vi "setPosition_fw103_wait.vi"(8 "waitTimeout":i32=500, 9 "Set position\n(deg) (float)":dbl, 11 "Method reference input":refnum<k24>) -> (1 "Current position (deg) (float)":i32 format="%.3f", 2 "error out":errorcluster, 3 "Method reference out":refnum<k24>)   [LabVIEW 2020]
uses:
  C:/Users/OPMuser/Documents/labview/fw103/Thorlabs.MotionControl.Benchtop.StepperMotorCLI.dll
  Thorlabs.MotionControl.Benchtop.StepperMotorCLI.dll
  <vilib>/Utility/error.llb/Error Cluster From Error Code.vi
  <vilib>/ErrorRing/Error Ring.xnode
panel:
  # "Move filter wheel VI"
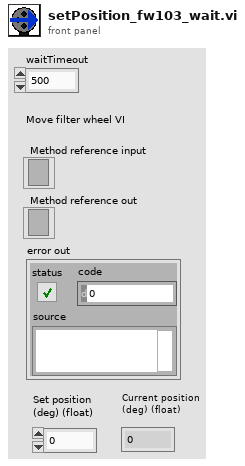
[diagram p1: front panel]
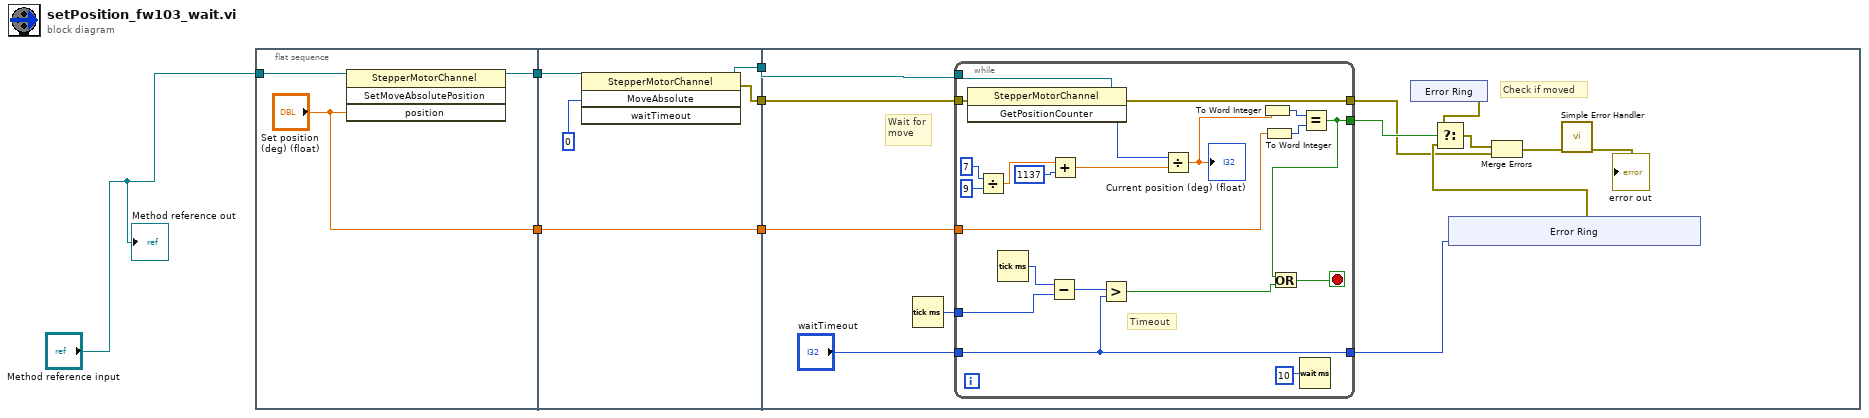
[diagram p0: block diagram]
diagram:
  n1 = flat-sequence {
    tunnel: [w9] -> w6
    tunnel: ["Set position\n(deg) (float)"] -> w3
    tunnel: "Method reference input" -> [w7]
    tunnel: w6 -> [w13]
    tunnel: [w12] -> w5
    tunnel: [w11] -> w4
    tunnel: w3 -> [w11]
    tunnel: [w10] -> w1
    tunnel: w1 -> [w19]
    tunnel: w4 -> [w21]
    tunnel: w5 -> [w22]
    frame #0 {
      n2 = invoke class="StepperMotorChannel" method="SetMoveAbsolutePosition"(reference=w7, "position"="Set position\n(deg) (float)") -> (reference out=w9:refnum<k24>)  [unwired: 2 in, 3 out]
    }
    frame #1 {
      n3 = invoke class="StepperMotorChannel" method="MoveAbsolute"(reference=w13, "waitTimeout"=0) -> (reference out=w12:refnum<k24>, error out=w10:errorcluster)  [unwired: 2 in, 2 out]
    }
    frame #2 {
      # "Wait for\nmove"
      # "Check if moved"
      n4 = Tick Count (ms)() -> (millisecond timer value=w17:u32)
      n5 = while {
        tunnel: w22 -> [w47]
        tunnel: w21 -> [w39]
        tunnel: [w29] -> w20
        tunnel: w19 -> [w35]
        tunnel: [w34] -> w18
        tunnel: w17 -> [w32]
        tunnel: "waitTimeout" -> [w30]
        tunnel: [w30] -> w15
        stop <- w27 stop-if-true
        # "Timeout"
        n6 = invoke class="StepperMotorChannel" method="GetPositionCounter"(reference=w47, error in=w35) -> (error out=w34:errorcluster, "GetPositionCounter"=w41:i32)  [unwired: 1 in, 1 out]
        n7 = Divide(x=7, y=9) -> (x/y=w44:dbl)
        n8 = Tick Count (ms)() -> (millisecond timer value=w33:u32)
        n9 = Subtract(x=w33, y=w32) -> (x-y=w31:u32)
        n10 = Add(x=w44, y=1137) -> (x+y=w42:dbl)
        n11 = Greater?(x=w31, y=w30) -> (0:w28:bool)
        n12 = Divide(x=w41, y=w42) -> (x/y=w40:dbl)
        "Current position (deg) (float)" <- w40
        n13 = To Word Integer(number=w40) -> (16bit integer=w38:i16)
        n14 = To Word Integer(number=w39) -> (16bit integer=w37:i16)
        n15 = Wait (ms)(milliseconds to wait=u32 10) -> ()  [unwired: 1 out]
        n16 = Equal?(x=w38, y=w37) -> (x = y?=w29:bool)
        n17 = Or(x=w29, y=w28) -> (x .or. y?=w27:bool)
      }
      n18 = xnode "Error Ring"() -> ("error out"=w26:errorcluster)
      n19 = xnode "Error Ring"("parameter 0"=w15) -> ("error out"=w25:errorcluster)
      n20 = Select(t=w26, s=w20, f=w25) -> (s? t:f=w24:errorcluster)
      n21 = Merge Errors(w24, w18) -> (w23:errorcluster)
      "error out" <- w23
      n22 = call <vilib>:"Simple Error Handler.vi"("error in (no error)"=w23) -> ()  [unwired: 4 in, 5 out]
    }
  }
  "Method reference out" <- "Method reference input"
